vi "Sweep Sequencer.vi"(4 "Default Motor Parameters":T1={"position"=10000.0, "velocity"=10000.0, "acceleration"=100000.0, "deceleration"=100000.0, "accel. jerk"=1000000.0, "decel. jerk"=1000000.0}, 5 "Axis Array":refnum<k21>[](array[refnum])=["Axis 1", "Axis 2", "Axis 3", "Axis 4", "Axis 5", "Axis 6", "Axis 7", "Axis 8"], 6 "Loop counter in":i32, 7 "Max delay (ms)":u32=1000, 8 "error in (no error)":errorcluster, 10 "cts per rev":dbl=1000.0 format="%#_13g", 11 "Message Queue":refnum<queue>) -> (0 "error out":errorcluster)   [LabVIEW 2014]
uses:
  support/Message Queue/Message Cluster.ctl
  EMC API/EMC_Typedef_Motor_Parameters.ctl
  Typedef/Typedef_Motor_Message.ctl
  Globals/Global Stop.vi
  support/Message Queue/Message Queue.lvlib
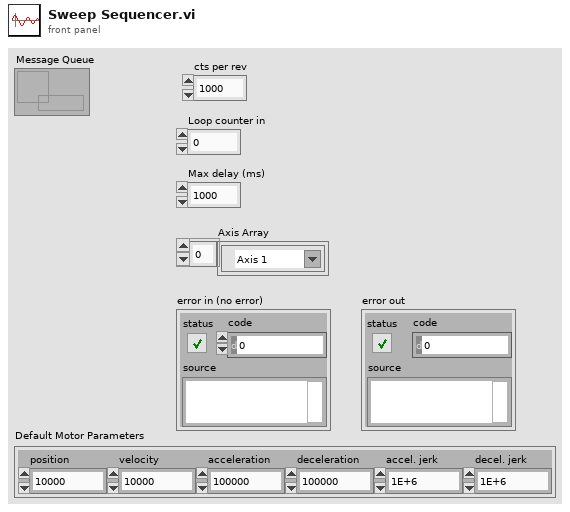
[diagram p1: front panel]
types:
  T1 = typedef "EMC_Typedef_Motor_Parameters.ctl" = cluster{"position":dbl, "velocity":dbl, "acceleration":dbl, "deceleration":dbl, "accel. jerk":dbl, "decel. jerk":dbl}
  T2 = typedef "Typedef_Motor_Message.ctl" = cluster{"Axis":refnum<k21>, "Motion Parameters":T1}
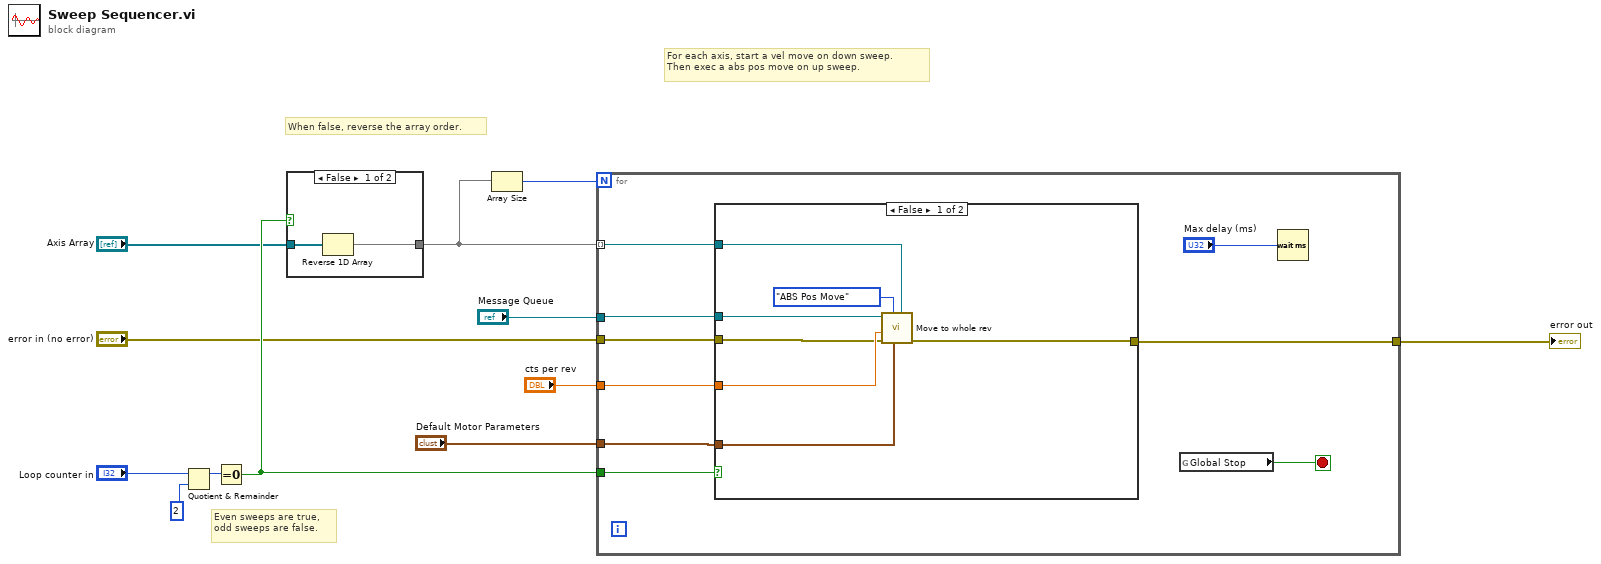
[diagram p0: block diagram]
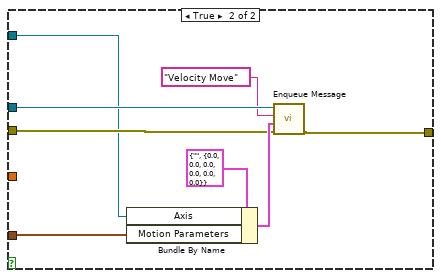
[diagram p3: hidden frame]
diagram:
  # "For each axis, start a vel move on down sweep.\nThen exec a abs pos move on up sweep."
  # "When false, reverse the array order."
  # "Even sweeps are true,\nodd sweeps are false."
  n1 = Quotient & Remainder(x="Loop counter in", y=2) -> (x-y*floor(x/y)=w11:i32)  [unwired: 1 out]
  n2 = Equal To 0?(x=w11) -> (x = 0?=w12:bool)
  n3 = case shown="False" w12 {
    tunnel: "Axis Array" -> [w14 w15]
    tunnel: [w13 w15] -> w5
    frame False {
      n4 = Reverse 1D Array(array=w14) -> (reversed array=w13:refnum<k21>[])
    }
    frame True {
    }
  }
  n5 = Array Size(array=w5) -> (size(s)=w6:i32)
  n6 = for {
    N: w6 -> [_]
    tunnel: [w17] -> w7
    tunnel: "Message Queue" -> [w21]
    tunnel: "error in (no error)" -> [w19]
    tunnel: w5 -> [w18] mode=indexing
    tunnel: w12 -> [w22]
    tunnel: "cts per rev" -> [w20]
    tunnel: "Default Motor Parameters" -> [w16]
    stop <- w23 stop-if-true
    n7 = case shown="False" w22 {
      tunnel: w21 -> [w30 w37]
      tunnel: w20 -> [w29 _]
      tunnel: w19 -> [w28 w36]
      tunnel: w18 -> [w27 w34]
      tunnel: [w26 w35] -> w17
      tunnel: w16 -> [w25 w32]
      frame False {
        n8 = call "Move to whole rev.vi"("resource in"=w27, "Default Motor Parameters"=w25, "Mode"=enum16{"ABS Pos Move", "REL Pos Move"}."ABS Pos Move", "error in (no error)"=w28, "cts per rev"=w29, "Queue in"=w30) -> ("error out"=w26:errorcluster)  [unwired: 4 in, 1 out]
      }
      frame True {
        n9 = Bundle By Name(cluster=T2 {"Axis"="", "Motion Parameters"={"position"=0.0, "velocity"=0.0, "acceleration"=0.0, "deceleration"=0.0, "accel. jerk"=0.0, "decel. jerk"=0.0}} ("Motor_Message"), "Axis"=w34, "Motion Parameters"=w32) -> (w39:T2)
        n10 = call "Enqueue Message.vi"("error in (no error)"=w36, "Message Data"=w39, "Message"="Velocity Move", "Message Queue"=w37) -> ("error out"=w35:errorcluster)  [unwired: 6 in, 1 out]
      }
    }
    n11 = global read "Global Stop.vi" "Global Stop"() -> (w23:bool)
    n12 = Wait (ms)(milliseconds to wait="Max delay (ms)") -> ()  [unwired: 1 out]
  }
  "error out" <- w7
